vi "Report Event.vi"(7 "Event Level (Info)":T1, 8 "error in (no error)":errorcluster, 10 "Message":string, 11 "EventLogHandler in":refnum<class "EventLogHandler.lvclass">) -> (0 "error out":errorcluster)   [LabVIEW 2020, in "Vecto.lvlib" / "EventLogHandler.lvclass"]
uses:
  EventLogHandler.lvclass
  Event Level.ctl
  Vecto.lvlib
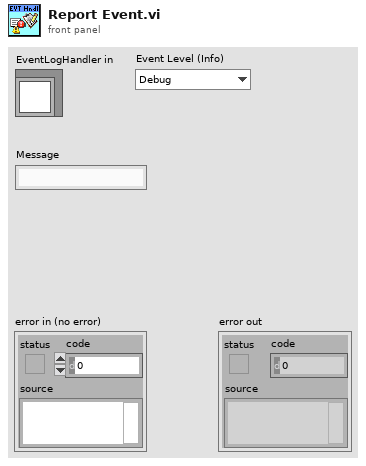
[diagram p1: front panel]
types:
  T1 = typedef "Vecto.lvlib/Event Level.ctl" = enum16{"Debug", "Info", "Warning", "Error"}
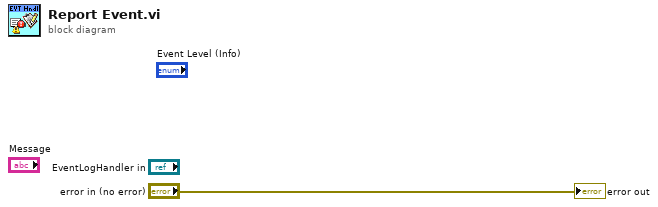
[diagram p0: block diagram]
diagram:
  "error out" <- "error in (no error)"
